vi "Send Error Status.vi"(10 "Errors":bool[](array[boolean])) -> ()   [LabVIEW 2020, in "Multiple Errors.lvclass"]
uses:
  Multiple Errors.lvclass
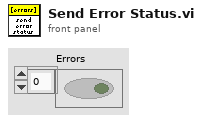
[diagram p1: front panel]
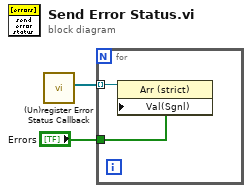
[diagram p0: block diagram]
diagram:
  n1 = call "(Un)register Error Status Callback.vi"() -> ("Registered controls"=w2:refnum<vi>[])  [unwired: 11 in]
  n2 = for {
    tunnel: w2 -> [w4] mode=indexing
    tunnel: "Errors" -> [w3]
    n3 = property class="Arr (strict)"(reference=w4, "Val(Sgnl)"=w3) -> ()  [unwired: 1 in, 2 out]
  }
